vi "Read DataGridViewNet.vi"(8 "error in (no error)":errorcluster, 11 "datagrid in":refnum<class "Data Grid.lvclass">) -> (0 "error out":errorcluster, 2 "DataGridView":refnum<k24>, 3 "datagrid out":refnum<class "Data Grid.lvclass">)   [LabVIEW 2015, in "Table Manager.lvlib" / "Data Grid.lvclass"]
uses:
  Data Grid.lvclass
  System.Windows.Forms
  Data Grid.lvclass/Data Grid.ctl
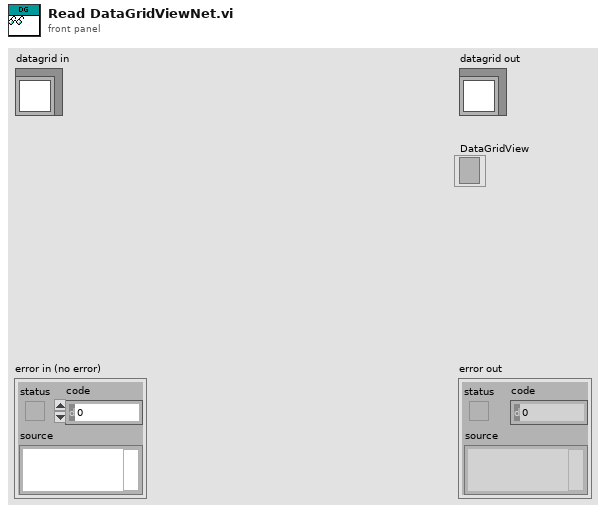
[diagram p1: front panel]
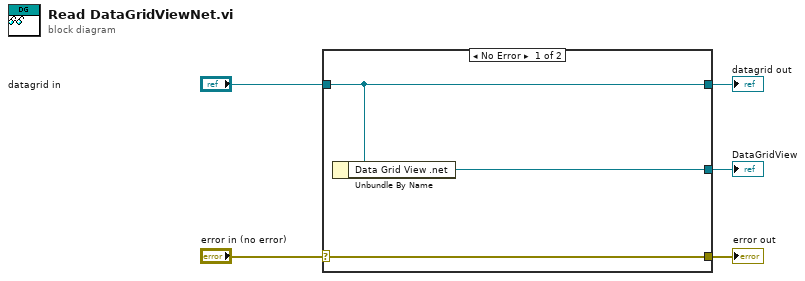
[diagram p0: block diagram]
diagram:
  n1 = case shown="No Error" "error in (no error)" {
    selector: "error in (no error)" -> [w8 w9]
    tunnel: [w8 w9] -> w4
    tunnel: [w7 w10] -> w2
    tunnel: "datagrid in" -> [w7 w10]
    tunnel: [w6 _] -> w1
    frame No Error {
      n2 = Unbundle By Name(w7) -> ("Data Grid View .net"=w6:refnum<k24>)
    }
    frame Error {
    }
  }
  "error out" <- w4
  "datagrid out" <- w2
  "DataGridView" <- w1
